vi "DBVar HandleOneElement.vi"(8 "error in (no error)":errorcluster, 10 "Terms":T1, 11 "Diagram":refnum<vi>) -> (0 "error out":errorcluster)   [LabVIEW 2012, in "NI_DB Variant To Data Support.lvlib"]
uses:
  NI_DB Variant To Data Support.lvlib
  <vilib>/XNodeSupport/XNodeTermIDPairs.ctl
  <vilib>/XNodeSupport/XNodeTermIDPair.ctl
  <vilib>/XNodeSupport/XNodeTermRef.ctl
  <vilib>/XNodeSupport/XNodeString.ctl
  <vilib>/XNodeSupport/NI_XNodeSupport.lvlib
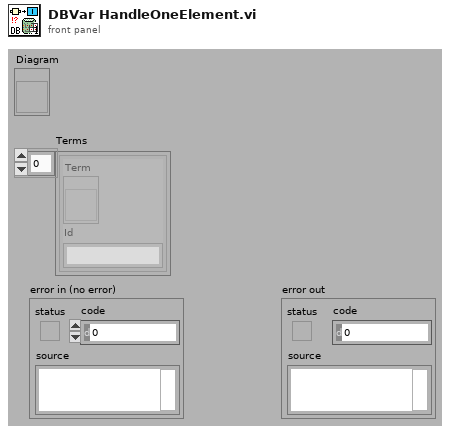
[diagram p1: front panel]
types:
  T1 = typedef "NI_XNodeSupport.lvlib/XNodeTermIDPairs.ctl" = T2[]
  T2 = typedef "NI_XNodeSupport.lvlib/XNodeTermIDPair.ctl" = cluster{"Term":T3, "Id":T4}
  T3 = typedef "NI_XNodeSupport.lvlib/XNodeTermRef.ctl" = refnum<vi>
  T4 = typedef "NI_XNodeSupport.lvlib/XNodeString.ctl" = string
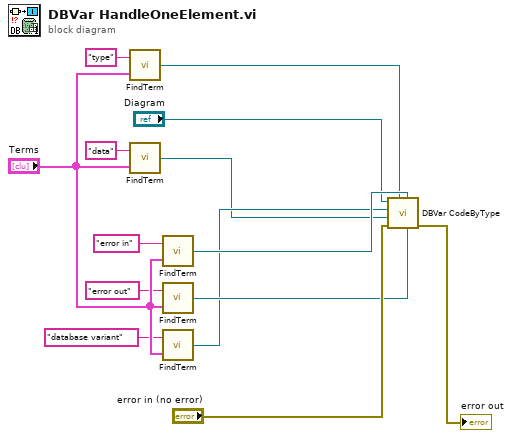
[diagram p0: block diagram]
diagram:
  n1 = call <vilib>:"FindTerm.vi"("Terms"="Terms", "String"="type") -> ("Term"=w1:refnum<vi>)
  n2 = call <vilib>:"FindTerm.vi"("Terms"="Terms", "String"="data") -> ("Term"=w2:refnum<vi>)
  n3 = call <vilib>:"FindTerm.vi"("Terms"="Terms", "String"="error in") -> ("Term"=w6:refnum<vi>)
  n4 = call <vilib>:"FindTerm.vi"("Terms"="Terms", "String"="error out") -> ("Term"=w5:refnum<vi>)
  n5 = call <vilib>:"FindTerm.vi"("Terms"="Terms", "String"="database variant") -> ("Term"=w3:refnum<vi>)
  n6 = call "DBVar CodeByType.vi"("Term error out"=w5, "Term error in"=w6, "Term type"=w1, "error in (no error)"="error in (no error)", "Term data out"=w2, "Term data in"=w3, "Diagram"="Diagram") -> ("error out"=→"error out":errorcluster)  [unwired: 4 in]
